vi "Clear.vi"(8 "error in (no error)":errorcluster, 11 "PQ Result  in":refnum<class "PQ Result.lvclass">) -> (0 "error out":errorcluster)   [LabVIEW 2015, in "PQ Result.lvclass"]
uses:
  PQ Result.lvclass
  PQ Result.lvclass/PQ Result.ctl
  <vilib>/LAVA/_libpq_internal_deps/libpq.dll
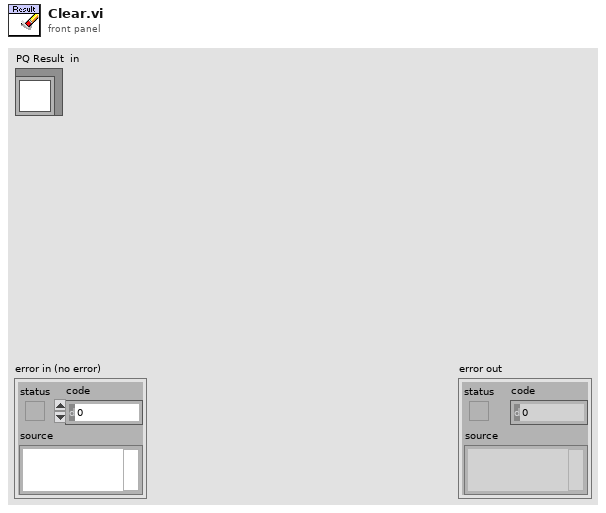
[diagram p1: front panel]
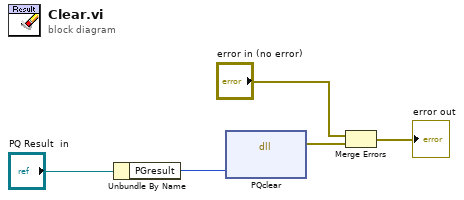
[diagram p0: block diagram]
diagram:
  n1 = Unbundle By Name("PQ Result  in") -> ("PGresult"=w2:u32)
  n2 = dll-call lib="C:/Program Files (x86)/National Instruments/LabVIEW 2015/vi.lib/LAVA/_libpq_internal_deps/libpq.dll" fn="PQclear"("PGresult"=w2) -> (error out=w1:errorcluster)  [unwired: 5 in, 1 out]
  n3 = Merge Errors("error in (no error)", w1) -> (→"error out":errorcluster)
